vi "Initialize Input DMA Refs.vi"(8 "error in (no error)":errorcluster, 10 "Settings.Compiled":T1 {"IncomingRegisters.Settings"."Register"."Data Type" format="%.0x"; "IncomingRegisters.Refs"."Refs"."Data Reference" format="%.0x"; "OutgoingRegisters.Settings"."Register"."Data Type" format="%.0x"; "OutgoingRegisters.Refs"."Refs"."Data Reference" format="%.0x"; "IncomingDMA.Settings"."Data Type" format="%.0x"; "IncomingDMA.Settings"."DMA.Settings"."DMA Host Buffer" items=["1 Second"=1, "2 Seconds"=2, "5 Seconds"=5, "10 Seconds"=10]; "IncomingDMA.Settings"."DMA.Settings"."dt" format="%#_p"; "IncomingDMA.Settings"."DMA.Settings"."Update Rate" items=["1 Hz"=1, "2 Hz"=2, "5 Hz"=5, "10 Hz"=10]; "OutgoingDMA.Settings"."Data Type" format="%.0x"; "OutgoingDMA.Settings"."DMA.Settings"."DMA Host Buffer" items=["1 Second"=1, "2 Seconds"=2, "5 Seconds"=5, "10 Seconds"=10]; "OutgoingDMA.Settings"."DMA.Settings"."dt" format="%#_p"; "OutgoingDMA.Settings"."DMA.Settings"."Update Rate" items=["1 Hz"=1, "2 Hz"=2, "5 Hz"=5, "10 Hz"=10]}, 11 "FPGA Ref":refnum<k20>) -> (0 "error out":errorcluster, 2 "DMA Settings":T15[](array[typedef]) {"Refs"."Data Type" format="%.0x"; "DMA Settings"."DMA Host Buffer" items=["1 Second"=1, "2 Seconds"=2, "5 Seconds"=5, "10 Seconds"=10]; "DMA Settings"."dt" format="%#_p"; "DMA Settings"."Update Rate" items=["1 Hz"=1, "2 Hz"=2, "5 Hz"=5, "10 Hz"=10]}, 3 "FPGA Ref":refnum<k20>)   [LabVIEW 2018, in "FPGA Addon Engine.lvlib"]
uses:
  FPGA Addon Engine.lvlib
  Types/DMA Input References.ctl
  <vilib>/NI Veristand/Custom Device Waveform API/Multiple Waveforms Write (DBL)/Multiple Waveforms Write (DBL).lvclass
  Addon Shared/Types/DMA Settings.ctl
  Addon Shared/Types/Delacing Scheme.ctl
  Addon Shared/Types/DMA Acquisition Mode.ctl
  Types/DMA Input Refs.ctl
  Addon Shared/Types/FPGA Addon Data Type.ctl
  Addon Shared/Types/Compiled.Settings.ctl
  Addon Shared/Types/Compiled.RegisterSettings.ctl
  Addon Shared/Types/Scalar Type.ctl
  Addon Shared/Types/Register Information.ctl
  <vilib>/NI Veristand/Custom Device API/Block Data Reference.ctl
  <vilib>/NI Veristand/Custom Device API/Data Reference.ctl
  Addon Shared/Types/Compiled.DMASettings.ctl
  <vilib>/NI Veristand/Custom Device API/Waveform Data Reference.ctl
  Addon Shared/Types/FPGA Settings.ctl
  <vilib>/NI Veristand/Custom Device API/Custom Device Target Type.ctl
  <vilib>/addons/FPGA Advanced Session Resources/LVFPGA Adv Session Resources/OpenByNameSubVI.vi
  <vilib>/rvi/interface/common/dynamic/niFpgaEscapeDelimiterAndNull.vi
  <vilib>/Utility/error.llb/Error Cluster From Error Code.vi
  <vilib>/rvi/interface/common/niFpgaWaitOnOcc.vi
  <vilib>/NI Veristand/Custom Device Waveform API/Multiple Waveforms Write (DBL)/NI VeriStand - Open Multiple Waveforms Write Session (DBL).vi
  <vilib>/addons/FPGA Advanced Session Resources/LVFPGA Adv Session Resources/OpenByName.xnode
  <vilib>/rvi/interface/nirviMethod/nirviMethod.xnode
  <vilib>/NI Veristand/Custom Device Waveform API/NI_VS Custom Device Waveform API.lvlib
  <vilib>/rvi/errors/niLvFpgaMergeErrorWithErrorCode.vi
  Addon Shared/FPGA Addon Shared.lvlib
  <vilib>/FPGAPlugInAG/Dynamic/niLvFpga_ConfigureFifo_Dynamic.vi
  <vilib>/FPGAPlugInAG/Dynamic/niLvFpga_StartFifo_Dynamic.vi
  <vilib>/addons/FPGA Advanced Session Resources/LVFPGA Adv Session Resources/LVFPGAAdvSessionResources.lvlib
  <vilib>/NI Veristand/Custom Device API/Custom Device API.lvlib
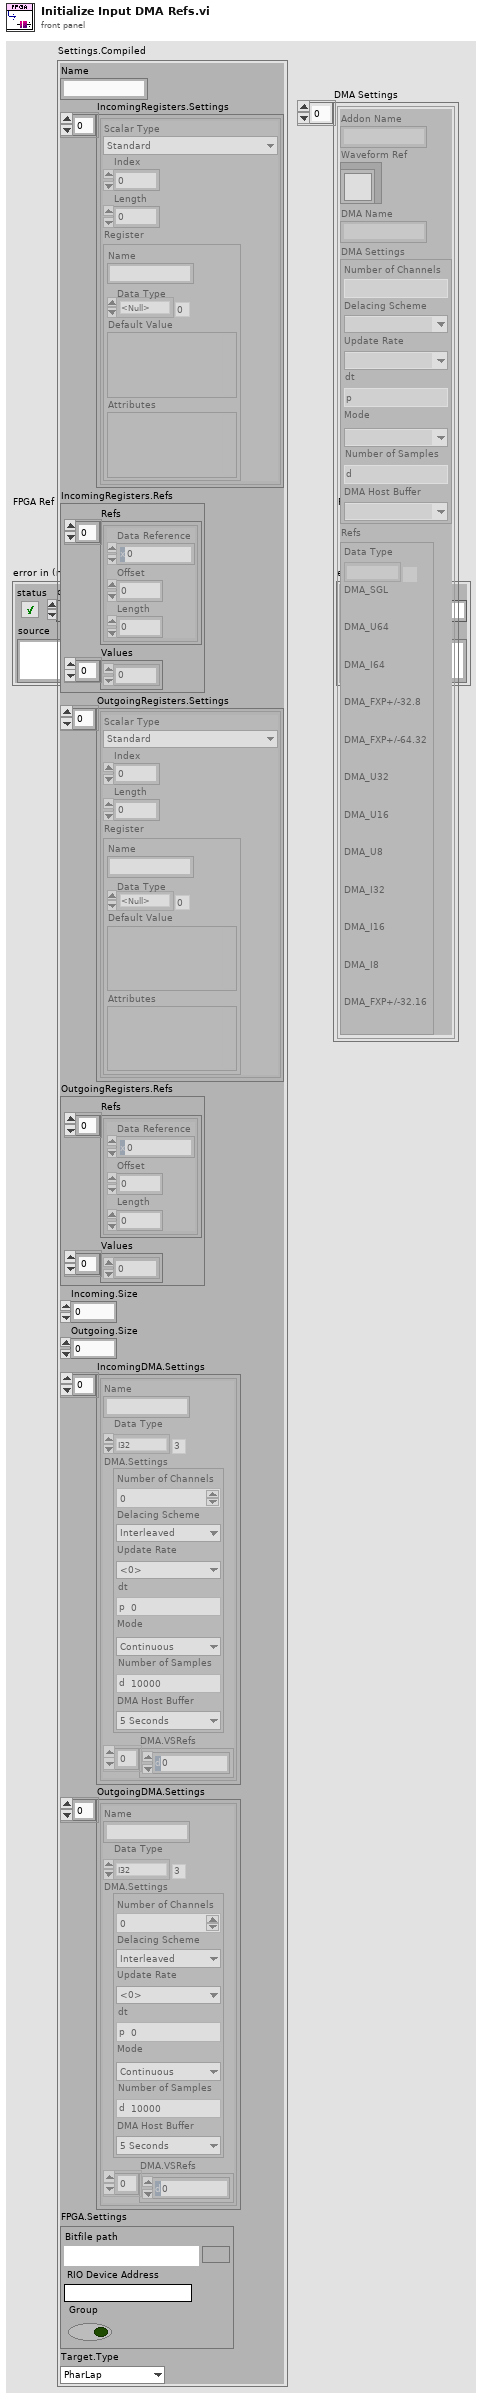
[diagram p1: front panel]
types:
  T1 = typedef "FPGA Addon Shared.lvlib/Compiled.Settings.ctl" = cluster{"Name":string, "IncomingRegisters.Settings":T2[], "IncomingRegisters.Refs":cluster{"Refs":T6[], "Values":dbl[]}, "OutgoingRegisters.Settings":T2[], "OutgoingRegisters.Refs":cluster{"Refs":T6[], "Values":dbl[]}, "Incoming.Size":i32, "Outgoing.Size":i32, "IncomingDMA.Settings":T8[], "OutgoingDMA.Settings":T8[], "FPGA.Settings":T13, "Target.Type":T14}
  T2 = typedef "FPGA Addon Shared.lvlib/Compiled.RegisterSettings.ctl" = cluster{"Scalar Type":T3, "Index":i32, "Length":i32, "Register":T4}
  T3 = typedef "FPGA Addon Shared.lvlib/Scalar Type.ctl" = enum16{"Standard", "Bitpacked"}
  T4 = typedef "FPGA Addon Shared.lvlib/Register Information.ctl" = cluster{"Name":string, "Data Type":T5, "Default Value":variant, "Attributes":variant}
  T5 = typedef "FPGA Addon Shared.lvlib/FPGA Addon Data Type.ctl" = enum8{"<Null>", "I8", "I16", "I32", "I64", "U8", "U16", "U32", "U64", "SGL", "Boolean", "Analog PWM In Settings", "Analog PWM In", "Digital PWM In Settings", "Digital PWM In", "Digital PWM Out", "Sine Out", "FXP", "FXP+/-24.5", "FXP+/-16.5", "FXP+/-32.8", "FXP+/-64.32", "FXP+/-16.7", "FXP+/-20.5", "FXP+/-27.5", "FXP+/-32.16", "FXP+16.3", "FXP+18.3", "Digital Static In", "Digital Static Out", "Digital Static In Settings", "Digital WSS Out", "Quad Encoder Settings", "Quad Encoder In", "Group"}
  T6 = typedef "Custom Device API.lvlib/Block Data Reference.ctl" = cluster{"Data Reference":T7, "Offset":u64, "Length":u64}
  T7 = typedef "Custom Device API.lvlib/Data Reference.ctl" = i32
  T8 = typedef "FPGA Addon Shared.lvlib/Compiled.DMASettings.ctl" = cluster{"Name":string, "Data Type":T5, "DMA.Settings":T9, "DMA.VSRefs":T12[]}
  T9 = typedef "FPGA Addon Shared.lvlib/DMA Settings.ctl" = cluster{"Number of Channels":u8, "Delacing Scheme":T10, "Update Rate":u32, "dt":dbl, "Mode":T11, "Number of Samples":u32, "DMA Host Buffer":u32}
  T10 = typedef "FPGA Addon Shared.lvlib/Delacing Scheme.ctl" = enum8{"Interleaved", "Bitpacked"}
  T11 = typedef "FPGA Addon Shared.lvlib/DMA Acquisition Mode.ctl" = enum8{"Continuous", "Triggered Finite"}
  T12 = typedef "Custom Device API.lvlib/Waveform Data Reference.ctl" = i32
  T13 = typedef "FPGA Addon Shared.lvlib/FPGA Settings.ctl" = cluster{"Bitfile path":path, "RIO Device Address":string, "Group":bool}
  T14 = typedef "Custom Device API.lvlib/Custom Device Target Type.ctl" = enum16{"PharLap", "VxWorks", "Windows", "Linux_32_ARM", "Linux_x64"}
  T15 = typedef "FPGA Addon Engine.lvlib/DMA Input References.ctl" = cluster{"Addon Name":string, "Waveform Ref":refnum<class "Multiple Waveforms Write (DBL).lvclass">, "DMA Name":string, "DMA Settings":T9, "Refs":T16}
  T16 = typedef "FPGA Addon Engine.lvlib/DMA Input Refs.ctl" = cluster{"Data Type":T5, "DMA_SGL":refnum<k20>, "DMA_U64":refnum<k20>, "DMA_I64":refnum<k20>, "DMA_FXP+/-32.8":refnum<k20>, "DMA_FXP+/-64.32":refnum<k20>, "DMA_U32":refnum<k20>, "DMA_U16":refnum<k20>, "DMA_U8":refnum<k20>, "DMA_I32":refnum<k20>, "DMA_I16":refnum<k20>, "DMA_I8":refnum<k20>, "DMA_FXP+/-32.16":refnum<k20>}
  T17 = cluster{"Name":string, "Depth":u32, "Write? (Deprecated:Use Implementation)":bool, "Physical Channel":u32, "Base Address":u32, "Data Width":u32, "Data Type":enum32{"Boolean", "I8", "I16", "I32", "I64", "U8", "U16", "U32", "U64", "FXP", "CustomControl", "SGL"}, "FXP Properties":variant, "Write Window Address":u32, "Implementation":enum16{"niFpgaTargetToHost", "niFpgaHostToTarget", "niFpgaPeerToPeerWriter", "niFpgaPeerToPeerReader", "niCoreTargetToHost", "niCoreHostToTarget"}, "Control Set":u32}[]
  T18 = cluster{"Name":string, "type":variant, "indicator?":bool}[]
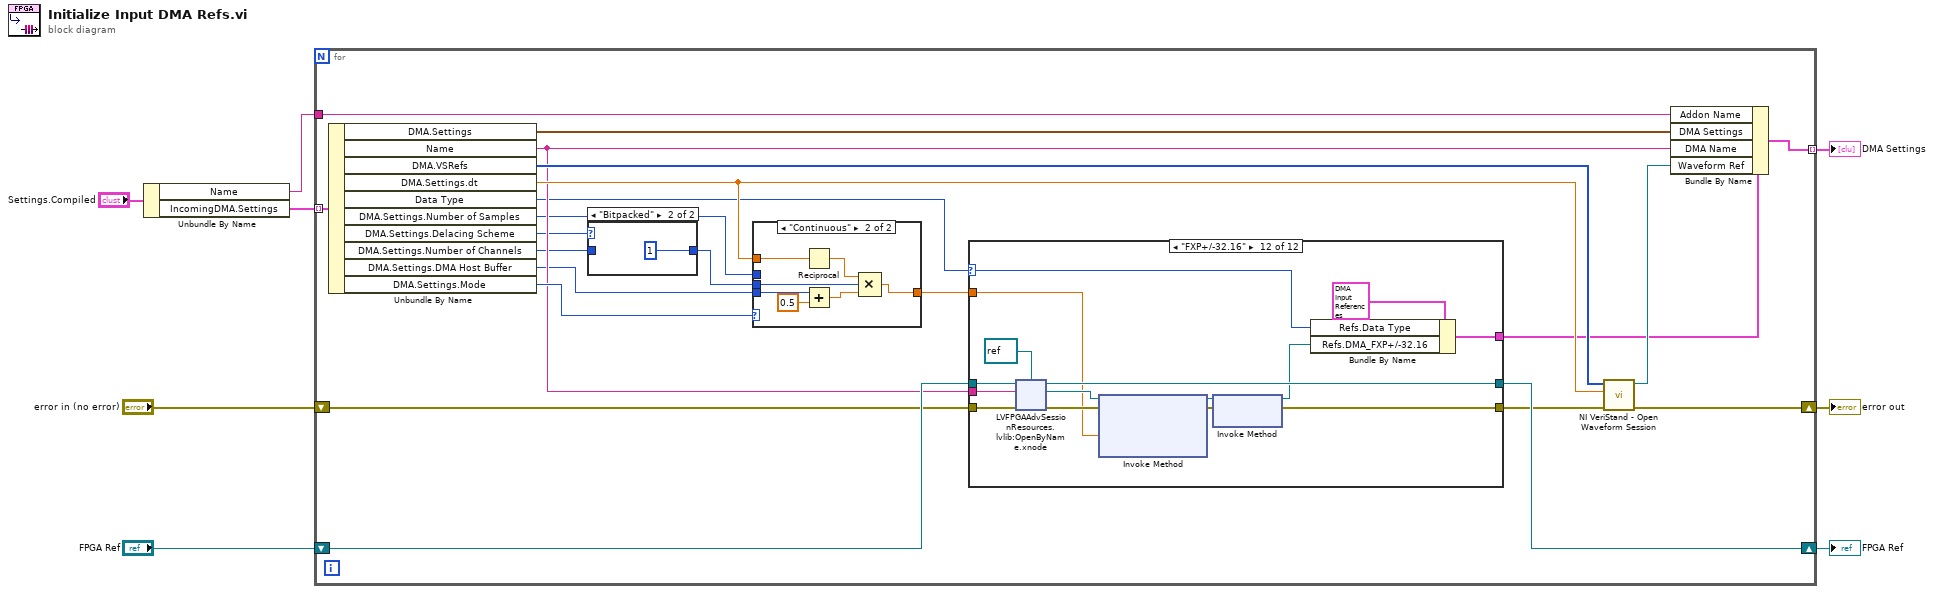
[diagram p0: block diagram]
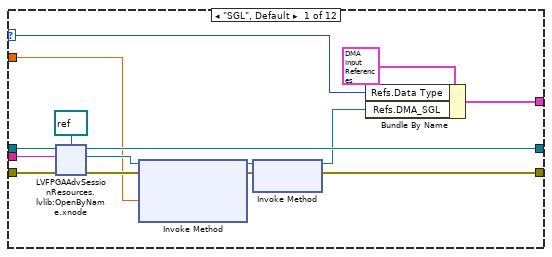
[diagram p3: hidden frame]
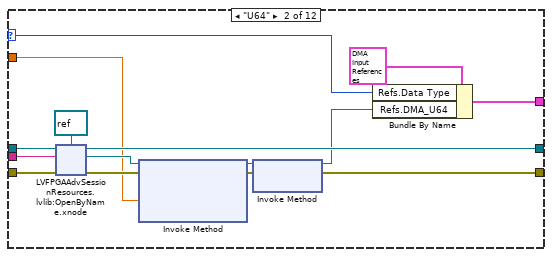
[diagram p4: hidden frame]
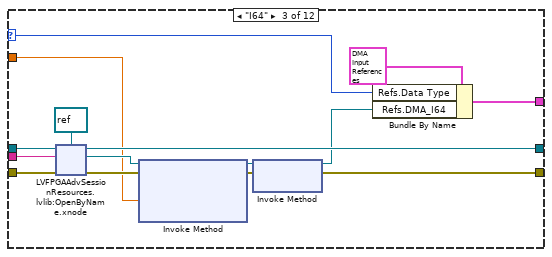
[diagram p5: hidden frame]
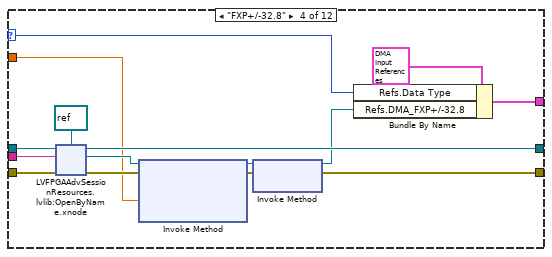
[diagram p6: hidden frame]
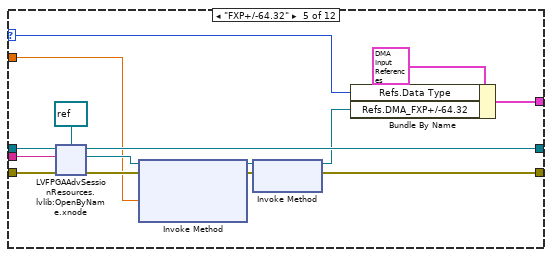
[diagram p7: hidden frame]
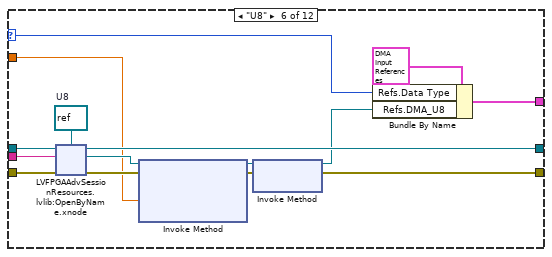
[diagram p8: hidden frame]
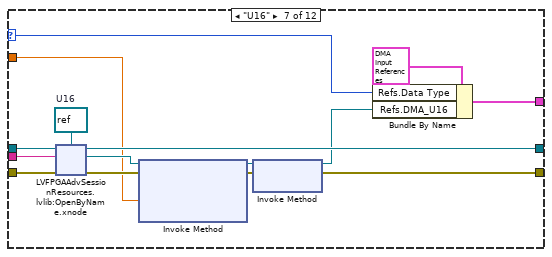
[diagram p9: hidden frame]
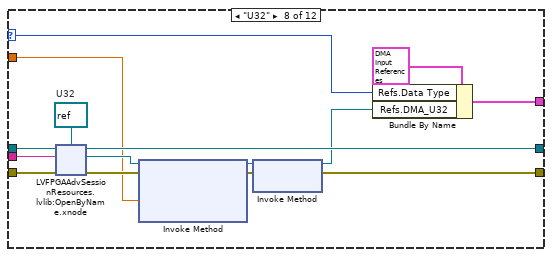
[diagram p10: hidden frame]
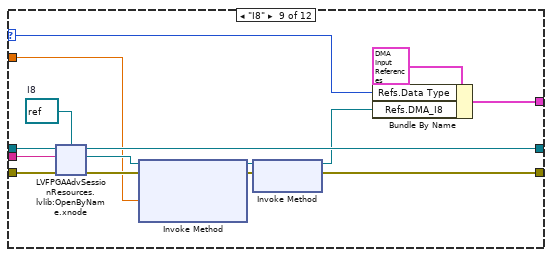
[diagram p11: hidden frame]
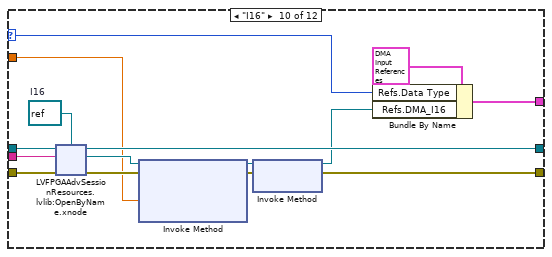
[diagram p12: hidden frame]
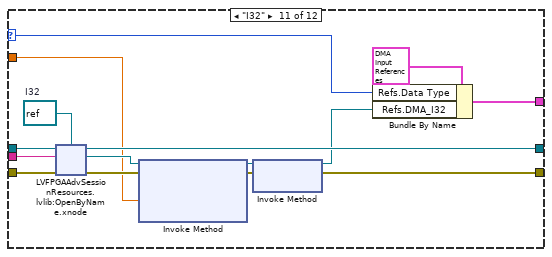
[diagram p13: hidden frame]
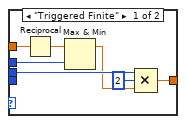
[diagram p14: hidden frame]
diagram:
  n1 = Unbundle By Name("Settings.Compiled") -> ("Name"=w1:string, "IncomingDMA.Settings"=w4:T8[])
  n2 = for {
    shift-right: [w29] -> w7
    shift-left: "FPGA Ref" -> [w30]
    tunnel: [w28] -> w6 mode=indexing
    tunnel: w4 -> [w25] mode=indexing
    shift-right: [w16] -> w3
    shift-left: "error in (no error)" -> [w23]
    tunnel: w1 -> [w9]
    n3 = Unbundle By Name(w25) -> ("DMA.Settings"=w20:T9, "Name"=w18:string, "DMA.VSRefs"=w22:T12[], "DMA.Settings.dt"=w26:dbl, "Data Type"=w13:T5, "DMA.Settings.Number of Samples"=w17:u32, "DMA.Settings.Delacing Scheme"=w12:T10, "DMA.Settings.Number of Channels"=w11:u8, "DMA.Settings.DMA Host Buffer"=w15:u32, "DMA.Settings.Mode"=w19:T11)
    n4 = case shown="\"Bitpacked\"" w12 {
      tunnel: [w31 u8 1 ("Number of Channels")] -> w10
      tunnel: w11 -> [w31 _]
      frame "Interleaved" {
      }
      frame "Bitpacked" {
      }
    }
    n5 = case shown="\"Continuous\"" w19 {
      tunnel: [w373 w382] -> w27
      tunnel: w26 -> [w372 w381]
      tunnel: w10 -> [w374 w380]
      tunnel: w17 -> [w370 _]
      tunnel: w15 -> [_ w379]
      frame "Triggered Finite" {
        n6 = Reciprocal(x=w372) -> (1/x=w371:dbl)
        n7 = Max & Min(x=w371, y=w370) -> (max(x,y)=w369:dbl)  [unwired: 1 out]
        n8 = Compound Arithmetic op=MULTIPLY(w374, u8 2 ("value"), w369) -> (w373:dbl)
      }
      frame "Continuous" {
        n9 = Reciprocal(x=w381) -> (1/x=w376:dbl)
        n10 = Add(x=w379, y=0.5 ("x")) -> (x+y=w378:dbl)
        n11 = Compound Arithmetic op=MULTIPLY(w376, w380, w378) -> (w382:dbl)
      }
    }
    n12 = case shown="\"FXP+/-32.16\"" w13 {
      selector: w13 -> [w33 w61 w90 w118 w146 w174 w202 w230 w258 w286 w314 w343]
      tunnel: w30 -> [w46 w75 w103 w131 w159 w187 w215 w243 w271 w299 w327 w355]
      tunnel: [w45 w74 w102 w130 w158 w186 w214 w242 w270 w298 w326 w354] -> w29
      tunnel: w27 -> [w40 w69 w97 w125 w153 w181 w209 w237 w265 w293 w321 w349]
      tunnel: [w39 w68 w96 w124 w152 w180 w208 w236 w264 w292 w320 w348] -> w24
      tunnel: w23 -> [w38 w67 w95 w123 w151 w179 w207 w235 w263 w291 w319 w347]
      tunnel: w18 -> [w37 w66 w94 w122 w150 w178 w206 w234 w262 w290 w318 w346]
      tunnel: [w34 w62 w91 w119 w147 w175 w203 w231 w259 w287 w315 w344] -> w14
      frame "SGL", Default {
        n13 = xnode "LVFPGAAdvSessionResources.lvlib:OpenByName.xnode"("FPGA VI Reference in"=w46, "Resource name in"=w37, "Single resource reference type in"=refnum<k20> refnum, "Error in"=w38) -> ("Single resource reference out"=w41:refnum<k20>, "Error out"=w42:errorcluster, "FPGA VI Reference out"=w45:refnum<k20>)
        n14 = xnode "Invoke Method"("FPGA VI Reference In"=w41, "error in"=w42, "Requested Depth"=w40) -> ("FPGA VI Reference Out"=w44:refnum<k20>, "error out"=w43:errorcluster)  [unwired: 1 out]
        n15 = xnode "Invoke Method"("FPGA VI Reference In"=w44, "error in"=w43) -> ("FPGA VI Reference Out"=w35:refnum<k20>, "error out"=w39:errorcluster)
        n16 = Bundle By Name(cluster=T15 {"Addon Name"="", "Waveform Ref"=refnum, "DMA Name"="", "DMA Settings"={"Number of Channels"=0, "Delacing Scheme"=enum."Interleaved", "Update Rate"=0, "dt"=0.0, "Mode"=enum."Continuous", "Number of Samples"=10000, "DMA Host Buffer"=5}, "Refs"={"Data Type"=enum."I32", "DMA_SGL"=refnum, "DMA_U64"=refnum, "DMA_I64"=refnum, "DMA_FXP+/-32.8"=refnum, "DMA_FXP+/-64.32"=refnum, "DMA_U32"=refnum, "DMA_U16"=refnum, "DMA_U8"=refnum, "DMA_I32"=refnum, "DMA_I16"=refnum, "DMA_I8"=refnum, "DMA_FXP+/-32.16"=refnum}}, "Refs.Data Type"=w33, "Refs.DMA_SGL"=w35) -> (w34:T15)
      }
      frame "U64" {
        n17 = xnode "LVFPGAAdvSessionResources.lvlib:OpenByName.xnode"("FPGA VI Reference in"=w75, "Resource name in"=w66, "Single resource reference type in"=refnum<k20> refnum, "Error in"=w67) -> ("Single resource reference out"=w70:refnum<k20>, "Error out"=w71:errorcluster, "FPGA VI Reference out"=w74:refnum<k20>)
        n18 = xnode "Invoke Method"("FPGA VI Reference In"=w70, "error in"=w71, "Requested Depth"=w69) -> ("FPGA VI Reference Out"=w73:refnum<k20>, "error out"=w72:errorcluster)  [unwired: 1 out]
        n19 = xnode "Invoke Method"("FPGA VI Reference In"=w73, "error in"=w72) -> ("FPGA VI Reference Out"=w64:refnum<k20>, "error out"=w68:errorcluster)
        n20 = Bundle By Name(cluster=T15 {"Addon Name"="", "Waveform Ref"=refnum, "DMA Name"="", "DMA Settings"={"Number of Channels"=0, "Delacing Scheme"=enum."Interleaved", "Update Rate"=0, "dt"=0.0, "Mode"=enum."Continuous", "Number of Samples"=10000, "DMA Host Buffer"=5}, "Refs"={"Data Type"=enum."I32", "DMA_SGL"=refnum, "DMA_U64"=refnum, "DMA_I64"=refnum, "DMA_FXP+/-32.8"=refnum, "DMA_FXP+/-64.32"=refnum, "DMA_U32"=refnum, "DMA_U16"=refnum, "DMA_U8"=refnum, "DMA_I32"=refnum, "DMA_I16"=refnum, "DMA_I8"=refnum, "DMA_FXP+/-32.16"=refnum}}, "Refs.Data Type"=w61, "Refs.DMA_U64"=w64) -> (w62:T15)
      }
      frame "I64" {
        n21 = xnode "LVFPGAAdvSessionResources.lvlib:OpenByName.xnode"("FPGA VI Reference in"=w103, "Resource name in"=w94, "Single resource reference type in"=refnum<k20> refnum ("DMA_I64"), "Error in"=w95) -> ("Single resource reference out"=w98:refnum<k20>, "Error out"=w99:errorcluster, "FPGA VI Reference out"=w102:refnum<k20>)
        n22 = xnode "Invoke Method"("FPGA VI Reference In"=w98, "error in"=w99, "Requested Depth"=w97) -> ("FPGA VI Reference Out"=w101:refnum<k20>, "error out"=w100:errorcluster)  [unwired: 1 out]
        n23 = xnode "Invoke Method"("FPGA VI Reference In"=w101, "error in"=w100) -> ("FPGA VI Reference Out"=w92:refnum<k20>, "error out"=w96:errorcluster)
        n24 = Bundle By Name(cluster=T15 {"Addon Name"="", "Waveform Ref"=refnum, "DMA Name"="", "DMA Settings"={"Number of Channels"=0, "Delacing Scheme"=enum."Interleaved", "Update Rate"=0, "dt"=0.0, "Mode"=enum."Continuous", "Number of Samples"=10000, "DMA Host Buffer"=5}, "Refs"={"Data Type"=enum."I32", "DMA_SGL"=refnum, "DMA_U64"=refnum, "DMA_I64"=refnum, "DMA_FXP+/-32.8"=refnum, "DMA_FXP+/-64.32"=refnum, "DMA_U32"=refnum, "DMA_U16"=refnum, "DMA_U8"=refnum, "DMA_I32"=refnum, "DMA_I16"=refnum, "DMA_I8"=refnum, "DMA_FXP+/-32.16"=refnum}}, "Refs.Data Type"=w90, "Refs.DMA_I64"=w92) -> (w91:T15)
      }
      frame "FXP+/-32.8" {
        n25 = xnode "LVFPGAAdvSessionResources.lvlib:OpenByName.xnode"("FPGA VI Reference in"=w131, "Resource name in"=w122, "Single resource reference type in"=refnum<k20> refnum ("FPGA Interface"), "Error in"=w123) -> ("Single resource reference out"=w126:refnum<k20>, "Error out"=w127:errorcluster, "FPGA VI Reference out"=w130:refnum<k20>)
        n26 = xnode "Invoke Method"("FPGA VI Reference In"=w126, "error in"=w127, "Requested Depth"=w125) -> ("FPGA VI Reference Out"=w129:refnum<k20>, "error out"=w128:errorcluster)  [unwired: 1 out]
        n27 = xnode "Invoke Method"("FPGA VI Reference In"=w129, "error in"=w128) -> ("FPGA VI Reference Out"=w120:refnum<k20>, "error out"=w124:errorcluster)
        n28 = Bundle By Name(cluster=T15 {"Addon Name"="", "Waveform Ref"=refnum, "DMA Name"="", "DMA Settings"={"Number of Channels"=0, "Delacing Scheme"=enum."Interleaved", "Update Rate"=0, "dt"=0.0, "Mode"=enum."Continuous", "Number of Samples"=10000, "DMA Host Buffer"=5}, "Refs"={"Data Type"=enum."I32", "DMA_SGL"=refnum, "DMA_U64"=refnum, "DMA_I64"=refnum, "DMA_FXP+/-32.8"=refnum, "DMA_FXP+/-64.32"=refnum, "DMA_U32"=refnum, "DMA_U16"=refnum, "DMA_U8"=refnum, "DMA_I32"=refnum, "DMA_I16"=refnum, "DMA_I8"=refnum, "DMA_FXP+/-32.16"=refnum}}, "Refs.Data Type"=w118, "Refs.DMA_FXP+/-32.8"=w120) -> (w119:T15)
      }
      frame "FXP+/-64.32" {
        n29 = xnode "LVFPGAAdvSessionResources.lvlib:OpenByName.xnode"("FPGA VI Reference in"=w159, "Resource name in"=w150, "Single resource reference type in"=refnum<k20> refnum ("FPGA Interface"), "Error in"=w151) -> ("Single resource reference out"=w154:refnum<k20>, "Error out"=w155:errorcluster, "FPGA VI Reference out"=w158:refnum<k20>)
        n30 = xnode "Invoke Method"("FPGA VI Reference In"=w154, "error in"=w155, "Requested Depth"=w153) -> ("FPGA VI Reference Out"=w157:refnum<k20>, "error out"=w156:errorcluster)  [unwired: 1 out]
        n31 = xnode "Invoke Method"("FPGA VI Reference In"=w157, "error in"=w156) -> ("FPGA VI Reference Out"=w148:refnum<k20>, "error out"=w152:errorcluster)
        n32 = Bundle By Name(cluster=T15 {"Addon Name"="", "Waveform Ref"=refnum, "DMA Name"="", "DMA Settings"={"Number of Channels"=0, "Delacing Scheme"=enum."Interleaved", "Update Rate"=0, "dt"=0.0, "Mode"=enum."Continuous", "Number of Samples"=10000, "DMA Host Buffer"=5}, "Refs"={"Data Type"=enum."I32", "DMA_SGL"=refnum, "DMA_U64"=refnum, "DMA_I64"=refnum, "DMA_FXP+/-32.8"=refnum, "DMA_FXP+/-64.32"=refnum, "DMA_U32"=refnum, "DMA_U16"=refnum, "DMA_U8"=refnum, "DMA_I32"=refnum, "DMA_I16"=refnum, "DMA_I8"=refnum, "DMA_FXP+/-32.16"=refnum}}, "Refs.Data Type"=w146, "Refs.DMA_FXP+/-64.32"=w148) -> (w147:T15)
      }
      frame "U8" {
        w173 = refnum<k20> refnum  # U8
        n33 = xnode "LVFPGAAdvSessionResources.lvlib:OpenByName.xnode"("FPGA VI Reference in"=w187, "Resource name in"=w178, "Single resource reference type in"=w173, "Error in"=w179) -> ("Single resource reference out"=w182:refnum<k20>, "Error out"=w183:errorcluster, "FPGA VI Reference out"=w186:refnum<k20>)
        n34 = xnode "Invoke Method"("FPGA VI Reference In"=w182, "error in"=w183, "Requested Depth"=w181) -> ("FPGA VI Reference Out"=w185:refnum<k20>, "error out"=w184:errorcluster)  [unwired: 1 out]
        n35 = xnode "Invoke Method"("FPGA VI Reference In"=w185, "error in"=w184) -> ("FPGA VI Reference Out"=w176:refnum<k20>, "error out"=w180:errorcluster)
        n36 = Bundle By Name(cluster=T15 {"Addon Name"="", "Waveform Ref"=refnum, "DMA Name"="", "DMA Settings"={"Number of Channels"=0, "Delacing Scheme"=enum."Interleaved", "Update Rate"=0, "dt"=0.0, "Mode"=enum."Continuous", "Number of Samples"=10000, "DMA Host Buffer"=5}, "Refs"={"Data Type"=enum."I32", "DMA_SGL"=refnum, "DMA_U64"=refnum, "DMA_I64"=refnum, "DMA_FXP+/-32.8"=refnum, "DMA_FXP+/-64.32"=refnum, "DMA_U32"=refnum, "DMA_U16"=refnum, "DMA_U8"=refnum, "DMA_I32"=refnum, "DMA_I16"=refnum, "DMA_I8"=refnum, "DMA_FXP+/-32.16"=refnum}}, "Refs.Data Type"=w174, "Refs.DMA_U8"=w176) -> (w175:T15)
      }
      frame "U16" {
        w201 = refnum<k20> refnum  # U16
        n37 = xnode "LVFPGAAdvSessionResources.lvlib:OpenByName.xnode"("FPGA VI Reference in"=w215, "Resource name in"=w206, "Single resource reference type in"=w201, "Error in"=w207) -> ("Single resource reference out"=w210:refnum<k20>, "Error out"=w211:errorcluster, "FPGA VI Reference out"=w214:refnum<k20>)
        n38 = xnode "Invoke Method"("FPGA VI Reference In"=w210, "error in"=w211, "Requested Depth"=w209) -> ("FPGA VI Reference Out"=w213:refnum<k20>, "error out"=w212:errorcluster)  [unwired: 1 out]
        n39 = xnode "Invoke Method"("FPGA VI Reference In"=w213, "error in"=w212) -> ("FPGA VI Reference Out"=w204:refnum<k20>, "error out"=w208:errorcluster)
        n40 = Bundle By Name(cluster=T15 {"Addon Name"="", "Waveform Ref"=refnum, "DMA Name"="", "DMA Settings"={"Number of Channels"=0, "Delacing Scheme"=enum."Interleaved", "Update Rate"=0, "dt"=0.0, "Mode"=enum."Continuous", "Number of Samples"=10000, "DMA Host Buffer"=5}, "Refs"={"Data Type"=enum."I32", "DMA_SGL"=refnum, "DMA_U64"=refnum, "DMA_I64"=refnum, "DMA_FXP+/-32.8"=refnum, "DMA_FXP+/-64.32"=refnum, "DMA_U32"=refnum, "DMA_U16"=refnum, "DMA_U8"=refnum, "DMA_I32"=refnum, "DMA_I16"=refnum, "DMA_I8"=refnum, "DMA_FXP+/-32.16"=refnum}}, "Refs.Data Type"=w202, "Refs.DMA_U16"=w204) -> (w203:T15)
      }
      frame "U32" {
        w229 = refnum<k20> refnum  # U32
        n41 = xnode "LVFPGAAdvSessionResources.lvlib:OpenByName.xnode"("FPGA VI Reference in"=w243, "Resource name in"=w234, "Single resource reference type in"=w229, "Error in"=w235) -> ("Single resource reference out"=w238:refnum<k20>, "Error out"=w239:errorcluster, "FPGA VI Reference out"=w242:refnum<k20>)
        n42 = xnode "Invoke Method"("FPGA VI Reference In"=w238, "error in"=w239, "Requested Depth"=w237) -> ("FPGA VI Reference Out"=w241:refnum<k20>, "error out"=w240:errorcluster)  [unwired: 1 out]
        n43 = xnode "Invoke Method"("FPGA VI Reference In"=w241, "error in"=w240) -> ("FPGA VI Reference Out"=w232:refnum<k20>, "error out"=w236:errorcluster)
        n44 = Bundle By Name(cluster=T15 {"Addon Name"="", "Waveform Ref"=refnum, "DMA Name"="", "DMA Settings"={"Number of Channels"=0, "Delacing Scheme"=enum."Interleaved", "Update Rate"=0, "dt"=0.0, "Mode"=enum."Continuous", "Number of Samples"=10000, "DMA Host Buffer"=5}, "Refs"={"Data Type"=enum."I32", "DMA_SGL"=refnum, "DMA_U64"=refnum, "DMA_I64"=refnum, "DMA_FXP+/-32.8"=refnum, "DMA_FXP+/-64.32"=refnum, "DMA_U32"=refnum, "DMA_U16"=refnum, "DMA_U8"=refnum, "DMA_I32"=refnum, "DMA_I16"=refnum, "DMA_I8"=refnum, "DMA_FXP+/-32.16"=refnum}}, "Refs.Data Type"=w230, "Refs.DMA_U32"=w232) -> (w231:T15)
      }
      frame "I8" {
        w257 = refnum<k20> refnum  # I8
        n45 = xnode "LVFPGAAdvSessionResources.lvlib:OpenByName.xnode"("FPGA VI Reference in"=w271, "Resource name in"=w262, "Single resource reference type in"=w257, "Error in"=w263) -> ("Single resource reference out"=w266:refnum<k20>, "Error out"=w267:errorcluster, "FPGA VI Reference out"=w270:refnum<k20>)
        n46 = xnode "Invoke Method"("FPGA VI Reference In"=w266, "error in"=w267, "Requested Depth"=w265) -> ("FPGA VI Reference Out"=w269:refnum<k20>, "error out"=w268:errorcluster)  [unwired: 1 out]
        n47 = xnode "Invoke Method"("FPGA VI Reference In"=w269, "error in"=w268) -> ("FPGA VI Reference Out"=w260:refnum<k20>, "error out"=w264:errorcluster)
        n48 = Bundle By Name(cluster=T15 {"Addon Name"="", "Waveform Ref"=refnum, "DMA Name"="", "DMA Settings"={"Number of Channels"=0, "Delacing Scheme"=enum."Interleaved", "Update Rate"=0, "dt"=0.0, "Mode"=enum."Continuous", "Number of Samples"=10000, "DMA Host Buffer"=5}, "Refs"={"Data Type"=enum."I32", "DMA_SGL"=refnum, "DMA_U64"=refnum, "DMA_I64"=refnum, "DMA_FXP+/-32.8"=refnum, "DMA_FXP+/-64.32"=refnum, "DMA_U32"=refnum, "DMA_U16"=refnum, "DMA_U8"=refnum, "DMA_I32"=refnum, "DMA_I16"=refnum, "DMA_I8"=refnum, "DMA_FXP+/-32.16"=refnum}}, "Refs.Data Type"=w258, "Refs.DMA_I8"=w260) -> (w259:T15)
      }
      frame "I16" {
        w285 = refnum<k20> refnum  # I16
        n49 = xnode "LVFPGAAdvSessionResources.lvlib:OpenByName.xnode"("FPGA VI Reference in"=w299, "Resource name in"=w290, "Single resource reference type in"=w285, "Error in"=w291) -> ("Single resource reference out"=w294:refnum<k20>, "Error out"=w295:errorcluster, "FPGA VI Reference out"=w298:refnum<k20>)
        n50 = xnode "Invoke Method"("FPGA VI Reference In"=w294, "error in"=w295, "Requested Depth"=w293) -> ("FPGA VI Reference Out"=w297:refnum<k20>, "error out"=w296:errorcluster)  [unwired: 1 out]
        n51 = xnode "Invoke Method"("FPGA VI Reference In"=w297, "error in"=w296) -> ("FPGA VI Reference Out"=w288:refnum<k20>, "error out"=w292:errorcluster)
        n52 = Bundle By Name(cluster=T15 {"Addon Name"="", "Waveform Ref"=refnum, "DMA Name"="", "DMA Settings"={"Number of Channels"=0, "Delacing Scheme"=enum."Interleaved", "Update Rate"=0, "dt"=0.0, "Mode"=enum."Continuous", "Number of Samples"=10000, "DMA Host Buffer"=5}, "Refs"={"Data Type"=enum."I32", "DMA_SGL"=refnum, "DMA_U64"=refnum, "DMA_I64"=refnum, "DMA_FXP+/-32.8"=refnum, "DMA_FXP+/-64.32"=refnum, "DMA_U32"=refnum, "DMA_U16"=refnum, "DMA_U8"=refnum, "DMA_I32"=refnum, "DMA_I16"=refnum, "DMA_I8"=refnum, "DMA_FXP+/-32.16"=refnum}}, "Refs.Data Type"=w286, "Refs.DMA_I16"=w288) -> (w287:T15)
      }
      frame "I32" {
        w313 = refnum<k20> refnum  # I32
        n53 = xnode "LVFPGAAdvSessionResources.lvlib:OpenByName.xnode"("FPGA VI Reference in"=w327, "Resource name in"=w318, "Single resource reference type in"=w313, "Error in"=w319) -> ("Single resource reference out"=w322:refnum<k20>, "Error out"=w323:errorcluster, "FPGA VI Reference out"=w326:refnum<k20>)
        n54 = xnode "Invoke Method"("FPGA VI Reference In"=w322, "error in"=w323, "Requested Depth"=w321) -> ("FPGA VI Reference Out"=w325:refnum<k20>, "error out"=w324:errorcluster)  [unwired: 1 out]
        n55 = xnode "Invoke Method"("FPGA VI Reference In"=w325, "error in"=w324) -> ("FPGA VI Reference Out"=w316:refnum<k20>, "error out"=w320:errorcluster)
        n56 = Bundle By Name(cluster=T15 {"Addon Name"="", "Waveform Ref"=refnum, "DMA Name"="", "DMA Settings"={"Number of Channels"=0, "Delacing Scheme"=enum."Interleaved", "Update Rate"=0, "dt"=0.0, "Mode"=enum."Continuous", "Number of Samples"=10000, "DMA Host Buffer"=5}, "Refs"={"Data Type"=enum."I32", "DMA_SGL"=refnum, "DMA_U64"=refnum, "DMA_I64"=refnum, "DMA_FXP+/-32.8"=refnum, "DMA_FXP+/-64.32"=refnum, "DMA_U32"=refnum, "DMA_U16"=refnum, "DMA_U8"=refnum, "DMA_I32"=refnum, "DMA_I16"=refnum, "DMA_I8"=refnum, "DMA_FXP+/-32.16"=refnum}}, "Refs.Data Type"=w314, "Refs.DMA_I32"=w316) -> (w315:T15)
      }
      frame "FXP+/-32.16" {
        n57 = xnode "LVFPGAAdvSessionResources.lvlib:OpenByName.xnode"("FPGA VI Reference in"=w355, "Resource name in"=w346, "Single resource reference type in"=refnum<k20> refnum ("Refs.DMA_FXP+/-32.16"), "Error in"=w347) -> ("Single resource reference out"=w350:refnum<k20>, "Error out"=w351:errorcluster, "FPGA VI Reference out"=w354:refnum<k20>)
        n58 = xnode "Invoke Method"("FPGA VI Reference In"=w350, "error in"=w351, "Requested Depth"=w349) -> ("FPGA VI Reference Out"=w353:refnum<k20>, "error out"=w352:errorcluster)  [unwired: 1 out]
        n59 = xnode "Invoke Method"("FPGA VI Reference In"=w353, "error in"=w352) -> ("FPGA VI Reference Out"=w341:refnum<k20>, "error out"=w348:errorcluster)
        n60 = Bundle By Name(cluster=T15 {"Addon Name"="", "Waveform Ref"=refnum, "DMA Name"="", "DMA Settings"={"Number of Channels"=0, "Delacing Scheme"=enum."Interleaved", "Update Rate"=0, "dt"=0.0, "Mode"=enum."Continuous", "Number of Samples"=10000, "DMA Host Buffer"=5}, "Refs"={"Data Type"=enum."I32", "DMA_SGL"=refnum, "DMA_U64"=refnum, "DMA_I64"=refnum, "DMA_FXP+/-32.8"=refnum, "DMA_FXP+/-64.32"=refnum, "DMA_U32"=refnum, "DMA_U16"=refnum, "DMA_U8"=refnum, "DMA_I32"=refnum, "DMA_I16"=refnum, "DMA_I8"=refnum, "DMA_FXP+/-32.16"=refnum}}, "Refs.Data Type"=w343, "Refs.DMA_FXP+/-32.16"=w341) -> (w344:T15)
      }
    }
    n61 = call-poly <vilib>:"NI VeriStand - Open Waveform Session.vi"("error in (no error)"=w24, "dt"=w26, "DBL Waveform Data References"=w22) -> ("error out"=w16:errorcluster, "Multiple Waveforms Write Session (DBL)"=w21:refnum<class "Multiple Waveforms Write (DBL).lvclass">)  [unwired: 7 in]
    n62 = Bundle By Name(cluster=w14, "Addon Name"=w9, "DMA Settings"=w20, "DMA Name"=w18, "Waveform Ref"=w21) -> (w28:T15)
  }
  "error out" <- w3
  "FPGA Ref" <- w7
  "DMA Settings" <- w6
